vi "Create.vi"(6 "timeout (-1)":i32=-1, 7 "EventDaemon in":refnum<class "TemplateDaemon.lvclass">, 8 "error in (no error)":errorcluster) -> (0 "error out":errorcluster, 3 "EventDaemon out":refnum<class "TemplateDaemon.lvclass">)   [LabVIEW 2024, in "TemplateDaemon.lvclass"]
doc: "Creates daemon class. By default, timeout is -1 and will wait for event messages. Set to millisecond delay time if a specific cycle time is required"
uses:
  TemplateDaemon.lvclass
  states--enum.ctl
  status--cluster.ctl
  TemplateDaemon.lvclass/TemplateDaemon.ctl
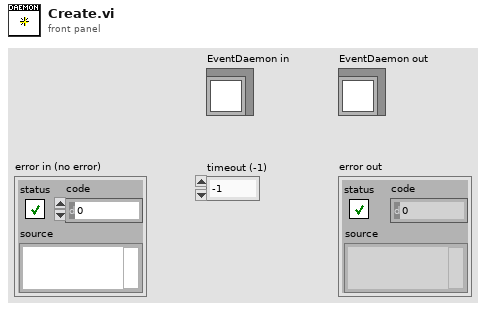
[diagram p1: front panel]
types:
  T1 = typedef "TemplateDaemon.lvclass/status--cluster.ctl" = cluster{"loop time":u32, "current state":T2, "error":errorcluster}
  T2 = typedef "TemplateDaemon.lvclass/states--enum.ctl" = enum16{"init", "default", "error handler", "exit"}
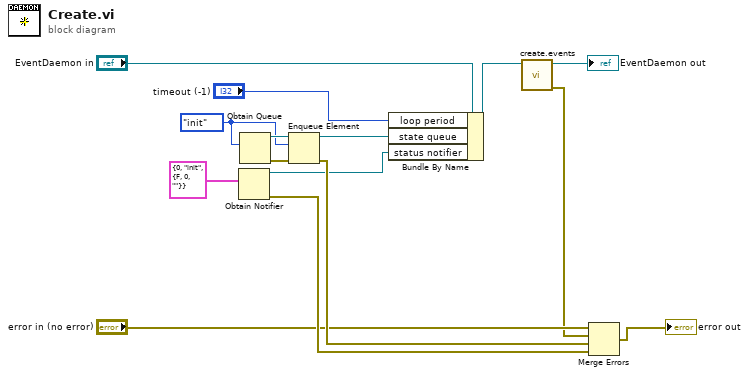
[diagram p0: block diagram]
diagram:
  w8 = states--enum."init" ("states")
  n1 = Obtain Notifier(notification data type=T1 {"loop time"=0, "current state"=enum."init", "error"={"status"=FALSE, "code"=0, "source"=""}} ("status")) -> (notifier out=w4:refnum<notifier>, error out=w3:errorcluster)  [unwired: 3 in, 1 out]
  n2 = Obtain Queue(element data type=w8) -> (queue out=w10:refnum<queue>, error out=w9:errorcluster)  [unwired: 4 in, 1 out]
  n3 = Enqueue Element(queue=w10, element=w8, error in (no error)=w9) -> (queue out=w7:refnum<queue>, error out=w6:errorcluster)  [unwired: 1 in, 1 out]
  n4 = Bundle By Name(cluster="EventDaemon in", "loop period"="timeout (-1)", "state queue"=w7, "status notifier"=w4) -> (w12:refnum<class "TemplateDaemon.lvclass">)
  n5 = call "create.events.vi"("EventDaemon in"=w12) -> ("error out"=w1:errorcluster, "EventDaemon out"=→"EventDaemon out":refnum<class "TemplateDaemon.lvclass">)  [unwired: 9 in]
  n6 = Merge Errors("error in (no error)", w1, w6, w3) -> (→"error out":errorcluster)
